vi "SetNoOfQuestion(SubVI).vi"() -> ()   [LabVIEW 2013]
uses:
  <vilib>/addons/database/Connection.llb/DB Tools Open Connec (String).vi
  <vilib>/addons/database/NI_Database_API.lvlib
panel:
  in  "Confirm&Back":bool
  in  "NoOfQn":dbl=15.0
  # "Please enter the number of questions you want to run. Default Value is 15."
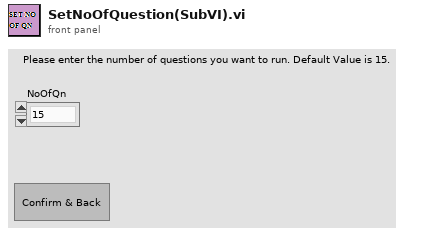
[diagram p1: front panel]
types:
  T1 = typedef "NI_Database_API.lvlib/Conn ObjectReference.ctl" = refnum<k1>
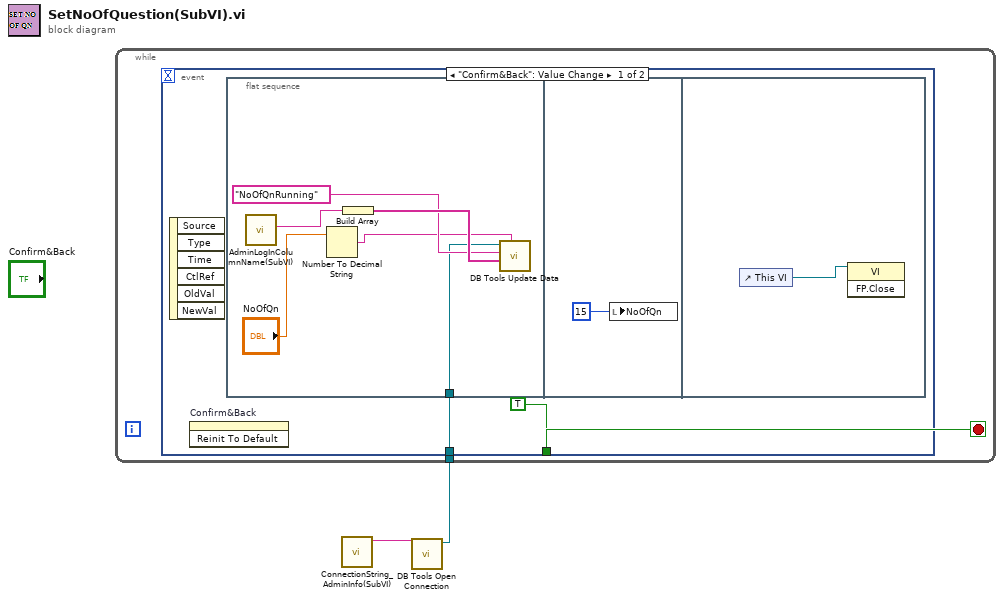
[diagram p0: block diagram]
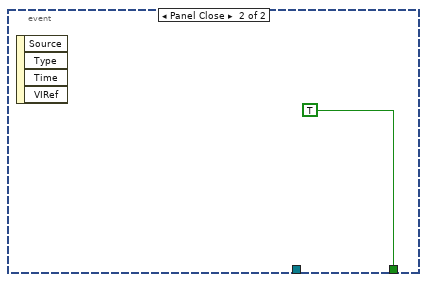
[diagram p2: hidden frame]
diagram:
  n1 = call "ConnectionString_AdminInfo(SubVI).vi"() -> ("ConnectionString"=w2:string)  [unwired: 11 in]
  n2 = call-poly <vilib>:"DB Tools Open Connection.vi"("connection information"=w2) -> ("connection reference"=w1:T1)  [unwired: 7 in, 1 out]
  n3 = while {
    tunnel: w1 -> [w3]
    stop <- w4 stop-if-true
    n4 = event shown="[0] \"Confirm&Back\": Value Change" {
      selector: _ -> [_ _]
      dyn-events: _ -> [_ _]
      timeout: _ -> [_ _]
      tunnel: [TRUE TRUE] -> w4
      tunnel: w3 -> [w5 _]
      event "Confirm&Back": Value Change {
        n5 = event-data() -> ()  [unwired: 1 in, 6 out]
        n6 = invoke on="Confirm&Back" class="Bool (strict)" method="Reinit To Default"() -> ()  [unwired: 3 in, 3 out]
        n7 = flat-sequence {
          tunnel: w5 -> [w8]
          frame #0 {
            n8 = call "AdminLogInColumnName(SubVI).vi"() -> ("Path for Score Table"=w9:string)  [unwired: 11 in]
            n9 = Number To Decimal String(number="NoOfQn") -> (decimal integer string=w10:string)  [unwired: 1 in]
            n10 = Build Array(w9) -> (w12:string[])
            n11 = call <vilib>:"DB Tools Update Data.vi"("data"=w10, "columns"=w12, "table"="NoOfQnRunning", "connection reference"=w8) -> ()  [unwired: 6 in, 2 out]
          }
          frame #1 {
            n12 = local write "NoOfQn"(15) -> ()
          }
          frame #2 {
            n13 = control-ref of="This VI"() -> (w14:refnum<vi>)
            n14 = invoke class="VI" method="FP.Close"(reference=w14) -> ()  [unwired: 2 in, 3 out]
          }
        }
      }
      event Panel Close {
        n15 = event-data() -> ()  [unwired: 1 in, 4 out]
      }
    }
  }
